vi "MSG Connect.vi"(8 "error in":errorcluster, 10 "Payload":variant) -> (0 "error out":errorcluster)   [LabVIEW 2020, in "Hardware.lvlib"]
uses:
  Hardware.lvlib
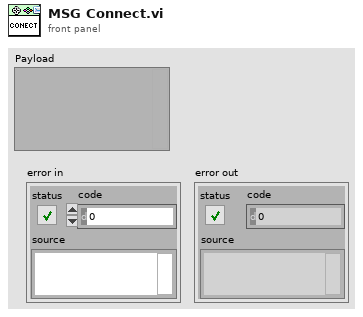
[diagram p1: front panel]
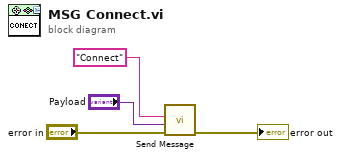
[diagram p0: block diagram]
diagram:
  n1 = call "Send Message.vi"("error in"="error in", "Payload"="Payload", "Command"="Connect") -> ("error out"=→"error out":errorcluster)  [unwired: 8 in]
